vi "Parse qLOG Answer.vi"(0 "Answer to Parse":string, 5 "error in":errorcluster) -> (14 "Array of LogInfo":T1[](array[typedef]) {"Error Code" min=1 max=4 step=1; "Index" min=1 max=4 step=1}, 19 "error out":errorcluster)   [LabVIEW 2020]
doc: "Parses the answer from the LOG? command.\n\nThis VI translates the UMF block answer from LOG? into an array of LogInfo.ctl elements."
uses:
  General command.llb/LogInfo.ctl
panel:
  # "Parses the answer from the LOG? command.\n\nThis VI translates the UMF block answer from LOG? into an array of LogInfo.ctl elements."
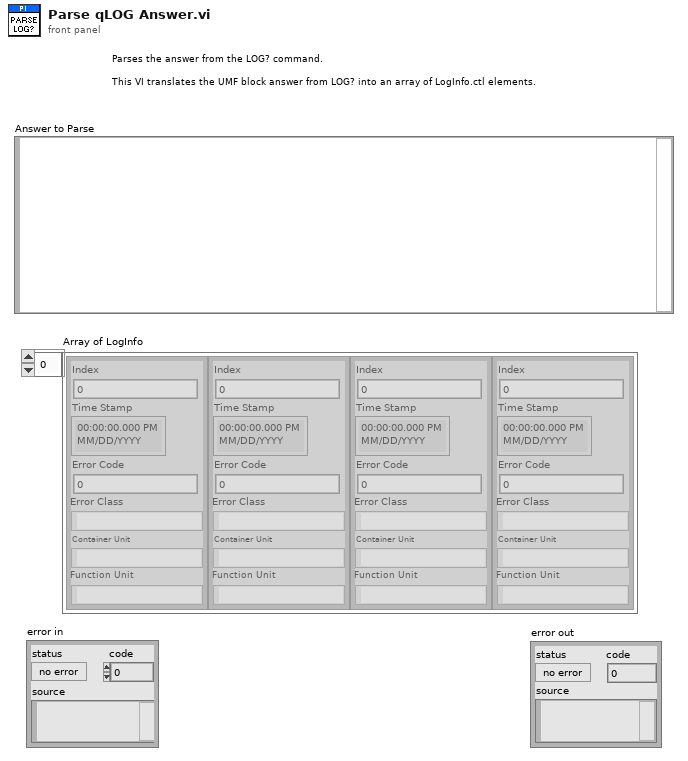
[diagram p1: front panel]
types:
  T1 = typedef "LogInfo.ctl" = cluster{"Index":i32, "Time Stamp":timestamp, "Error Code":i32, "Error Class":string, "Container Unit":string, "Function Unit":string}
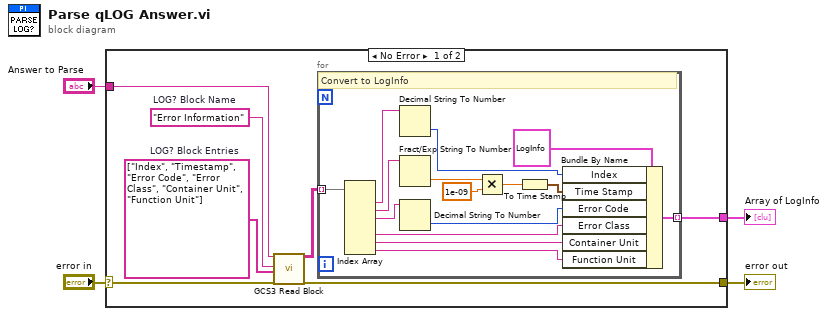
[diagram p0: block diagram]
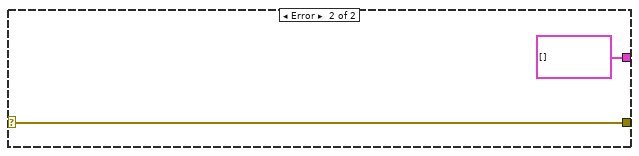
[diagram p2: hidden frame]
diagram:
  n1 = case shown="No Error" "error in" {
    selector: "error in" -> [w8 w28]
    tunnel: [w5 w28] -> w3
    tunnel: "Answer to Parse" -> [w11 _]
    tunnel: [w6 T1[] [] ("Array of LogInfo")] -> w1
    frame No Error {
      w9 = string[] ["Index", "Timestamp", "Error Code", "Error Class", "Container Unit", "Function Unit"]  # LOG? Block Entries
      w10 = "Error Information"  # LOG? Block Name
      n2 = call "GCS3 Read Block.vi"("GCS 3.0 Block to Parse"=w11, "Expected GCS 3.0 Block Name"=w10, "List of expected GCS 3.0 Block Entries"=w9, "error in"=w8) -> ("List of extracted GCS 3.0 Block Entries"=w7:string[][], "error out"=w5:errorcluster)  [unwired: 14 in]
      n3 = for {
        tunnel: w7 -> [w19] mode=indexing
        tunnel: [w17] -> w6 mode=indexing
        # "Convert to LogInfo"
        n4 = Index Array(array=w19) -> (element #1=w20:string, element #2=w13:string, element #3=w21:string, element #5=w16:string, element #6=w15:string, element #7=w14:string)  [unwired: 7 in, 1 out]
        n5 = Decimal String To Number(string=w20) -> (number=w25:i32)  [unwired: 2 in, 1 out]
        n6 = Fract/Exp String To Number(string=w13) -> (number=w12:dbl)  [unwired: 3 in, 1 out]
        n7 = Decimal String To Number(string=w21) -> (number=w18:i32)  [unwired: 2 in, 1 out]
        n8 = Multiply(x=w12, y=1e-09) -> (x*y=w22:dbl)
        n9 = To Time Stamp(1:w22) -> (0:w24:timestamp)
        n10 = Bundle By Name(cluster=T1 {"Index"=0, "Time Stamp"=timestamp(0 s since 1904-01-01), "Error Code"=0, "Error Class"="", "Container Unit"="", "Function Unit"=""} ("LogInfo"), "Index"=w25, "Time Stamp"=w24, "Error Code"=w18, "Error Class"=w16, "Container Unit"=w15, "Function Unit"=w14) -> (w17:T1)
      }
    }
    frame Error {
    }
  }
  "error out" <- w3
  "Array of LogInfo" <- w1
